vi "Reader kod10.vi"() -> ()   [LabVIEW 2021]
uses:
  <vilib>/Utility/file.llb/Write Delimited Spreadsheet (string).vi
  <vilib>/Utility/file.llb/Write Delimited Spreadsheet (DBL).vi
  <vilib>/FPGAPlugInAG/myRIO-1900/niLvFpga_Open_myRIO-1900.vi
  <vilib>/rvi/interface/common/dynamic/niFpgaDynamicAddResources.vi
  <vilib>/Utility/error.llb/Error Cluster From Error Code.vi
  <vilib>/rvi/errors/niLvFpgaAdjustHostInterfaceError.vi
  <vilib>/rvi/interface/nirviOpenFPGA/nirviOpenFPGA.xnode
  FPGA Bitfiles/projekt-bms10_FPGATarget_FPG10_wC+vpsaqoBo.lvbitx
  FPG10.vi
  <vilib>/rvi/interface/nirviReadWriteControl/nirviReadWriteControl.xnode
  <vilib>/rvi/interface/Simulation/niFpgaSimulationCallBeginRW.vi
  NiFpgaLv.dll
panel:
  out "Spänning 144 output 3":fxp<+/-,26,14>
  in  "stop 4":bool
  out "Loopar":fxp<+/-,64,32>
  out "SoC minus":fxp<+/-,32,16> format="%.21g"
  in  "stop 2":bool
  out "SoC":fxp<+/-,64,56>
  out "Batteri 2":fxp<+/-,64,54> format="%.21g"
  out "Ström 144 output":dbl format="%.2f"
  out "Spänning 144 output":fxp<+/-,64,50>
  out "x/y":fxp<+/-,49,33>
  out "PERIOD TIME [ms] 12":u32
  out "DUTY CYCLE [ticks] 12":u32
  out "duty cycle 12":dbl
  out "PERIOD TIME [ms] 11":u32
  out "DUTY CYCLE [ticks] 11":u32
  out "duty cycle 11":dbl
  out "PERIOD TIME [ms] 10":u32
  out "DUTY CYCLE [ticks] 10":u32
  out "duty cycle 6":dbl
  out "PERIOD TIME [ms] 9":u32
  out "DUTY CYCLE [ticks] 9":u32
  out "duty cycle 5":dbl
  out "PERIOD TIME [ms] 8":u32
  out "DUTY CYCLE [ticks] 8":u32
  out "duty cycle 10":dbl
  out "PERIOD TIME [ms] 7":u32
  out "DUTY CYCLE [ticks] 7":u32
  out "duty cycle 9":dbl
  out "PERIOD TIME [ms] 6":u32
  out "DUTY CYCLE [ticks] 6":u32
  out "duty cycle 4":dbl
  out "PERIOD TIME [ms] 5":u32
  out "DUTY CYCLE [ticks] 5":u32
  out "duty cycle 3":dbl
  out "PERIOD TIME [ms] 4":u32
  out "DUTY CYCLE [ticks] 4":u32
  out "duty cycle 8":dbl
  out "PERIOD TIME [ms] 3":u32
  out "DUTY CYCLE [ticks] 3":u32
  out "duty cycle 7":dbl
  out "PERIOD TIME [ms] 2":u32
  out "DUTY CYCLE [ticks] 2":u32
  out "duty cycle 2":dbl
  out "PERIOD TIME [ms]":u32
  out "DUTY CYCLE [ticks]":u32
  out "duty cycle":dbl format="%#.4f"
  in  "stop":bool
  out "appended array":dbl[][](array[numeric])
  in  "file path (dialog if empty)":path
  out "Array":string[](array[string])
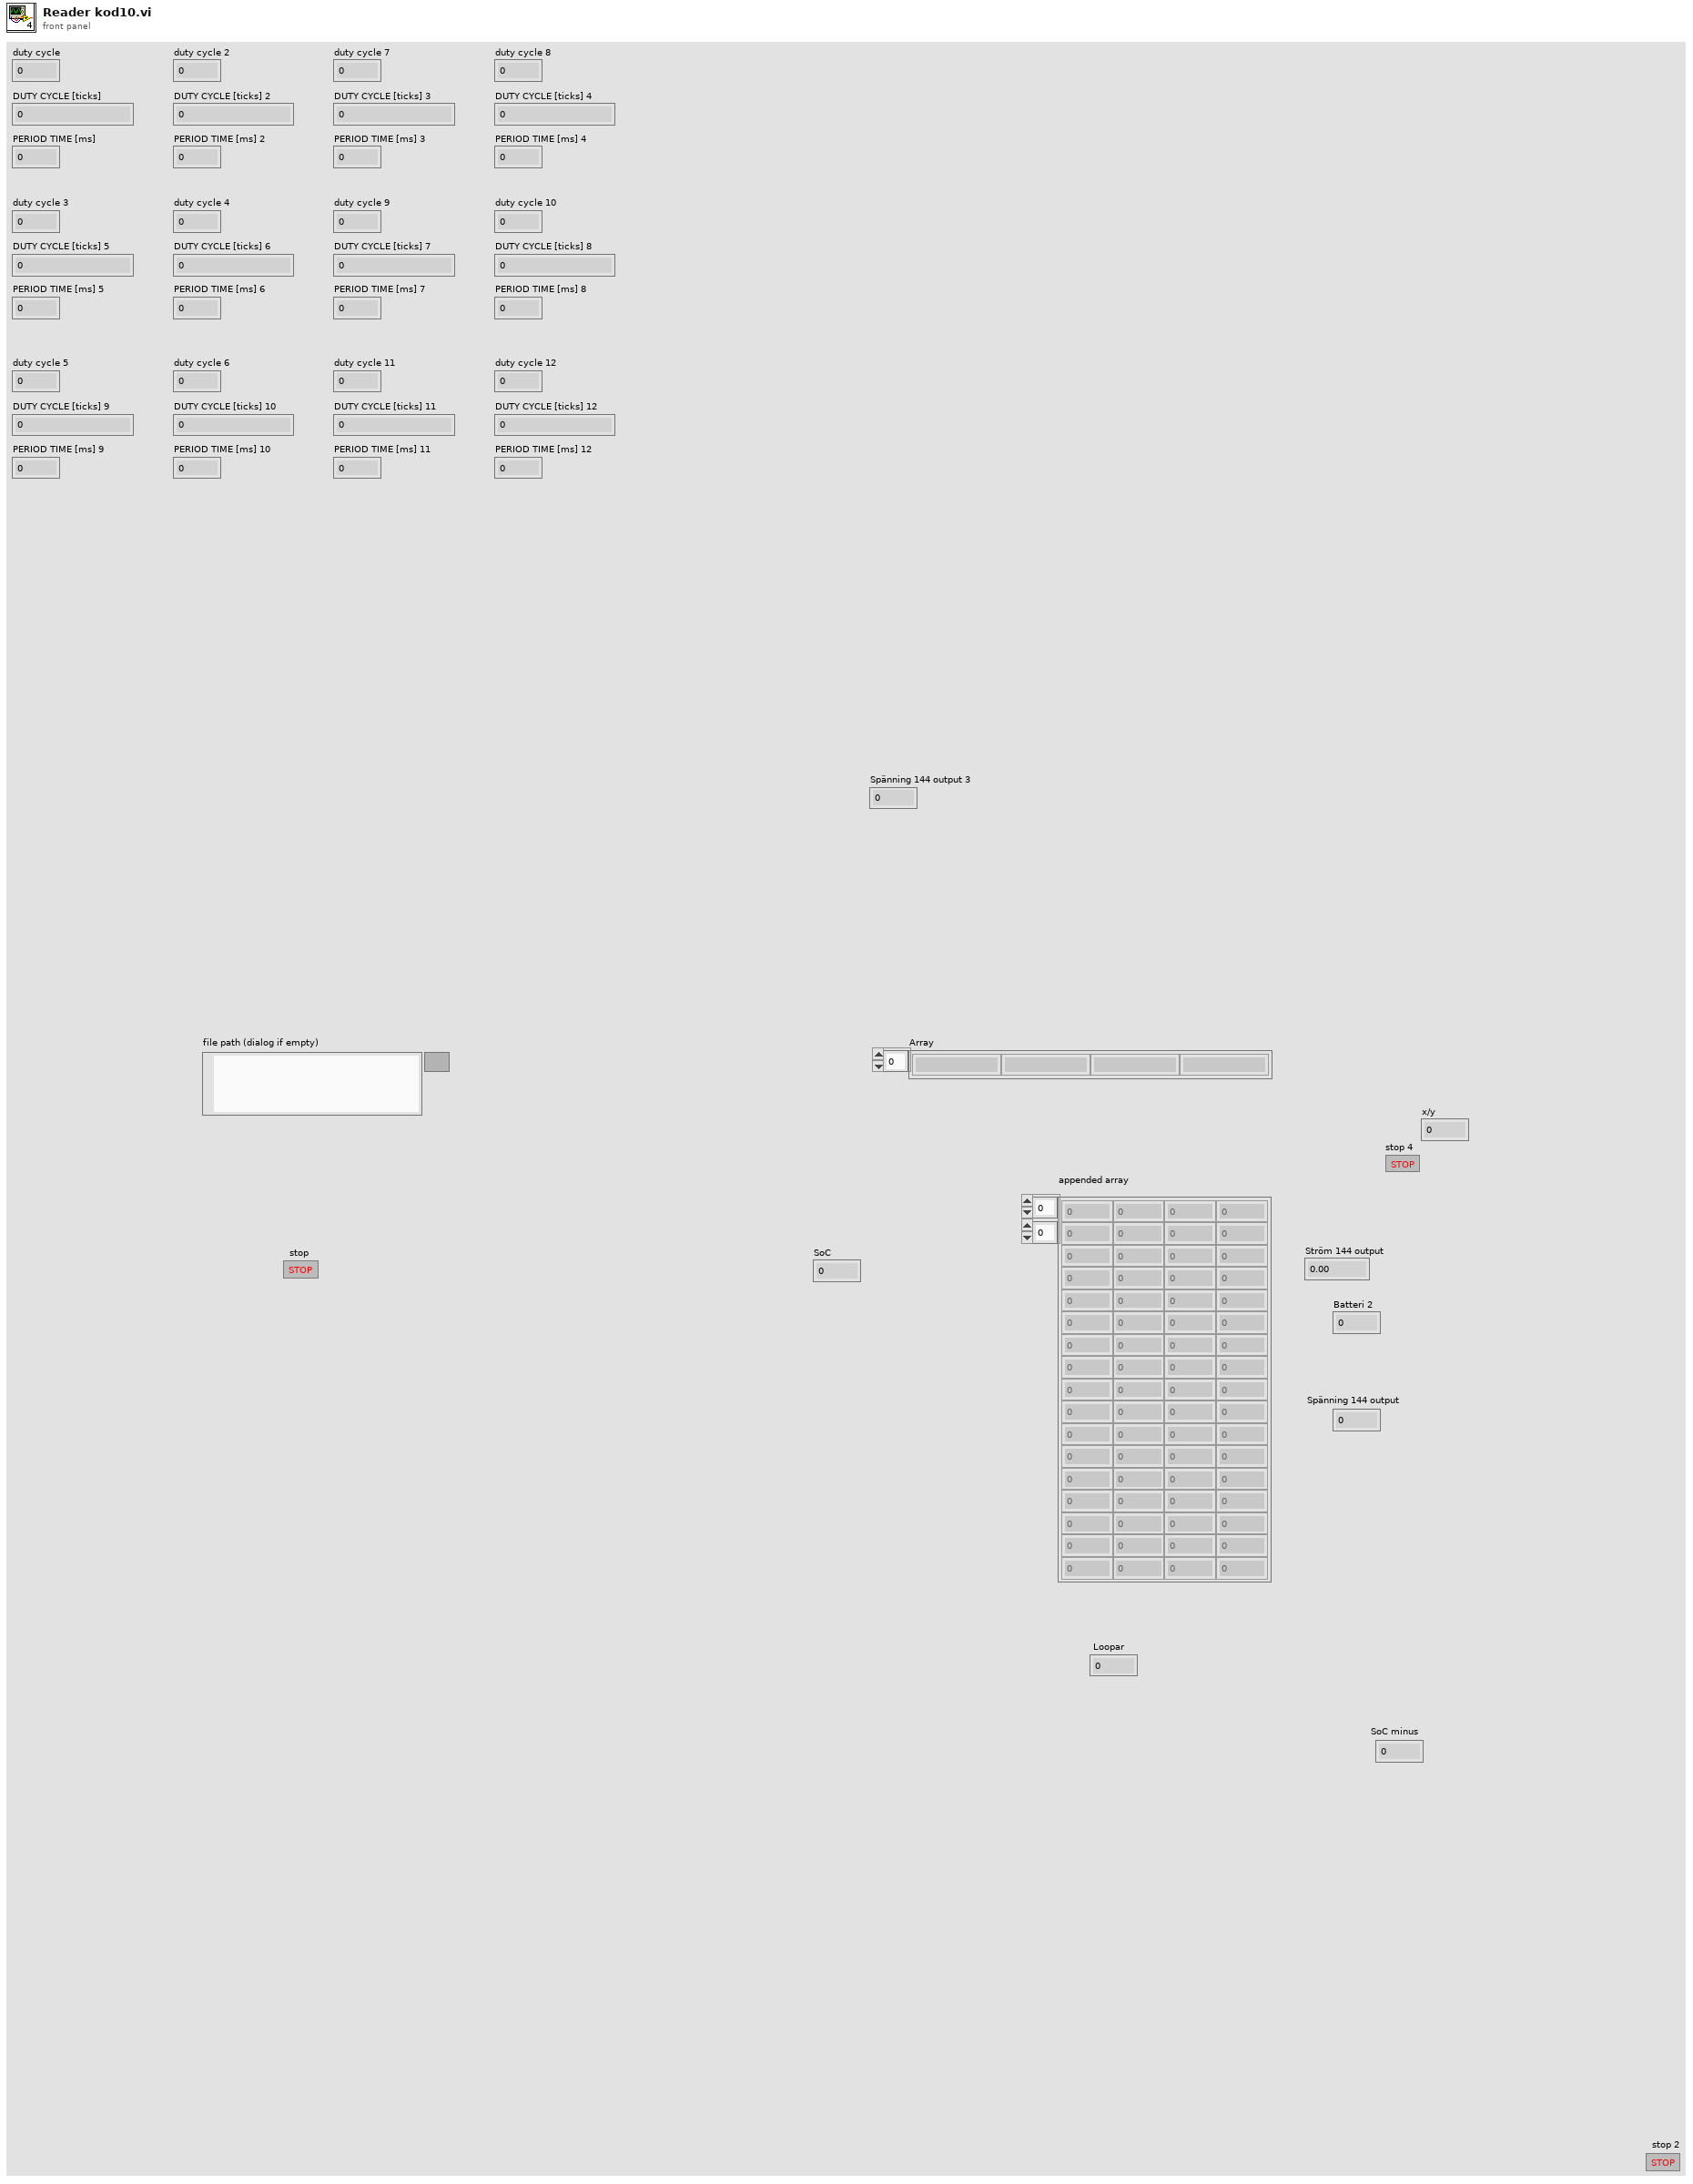
[diagram p1: front panel]
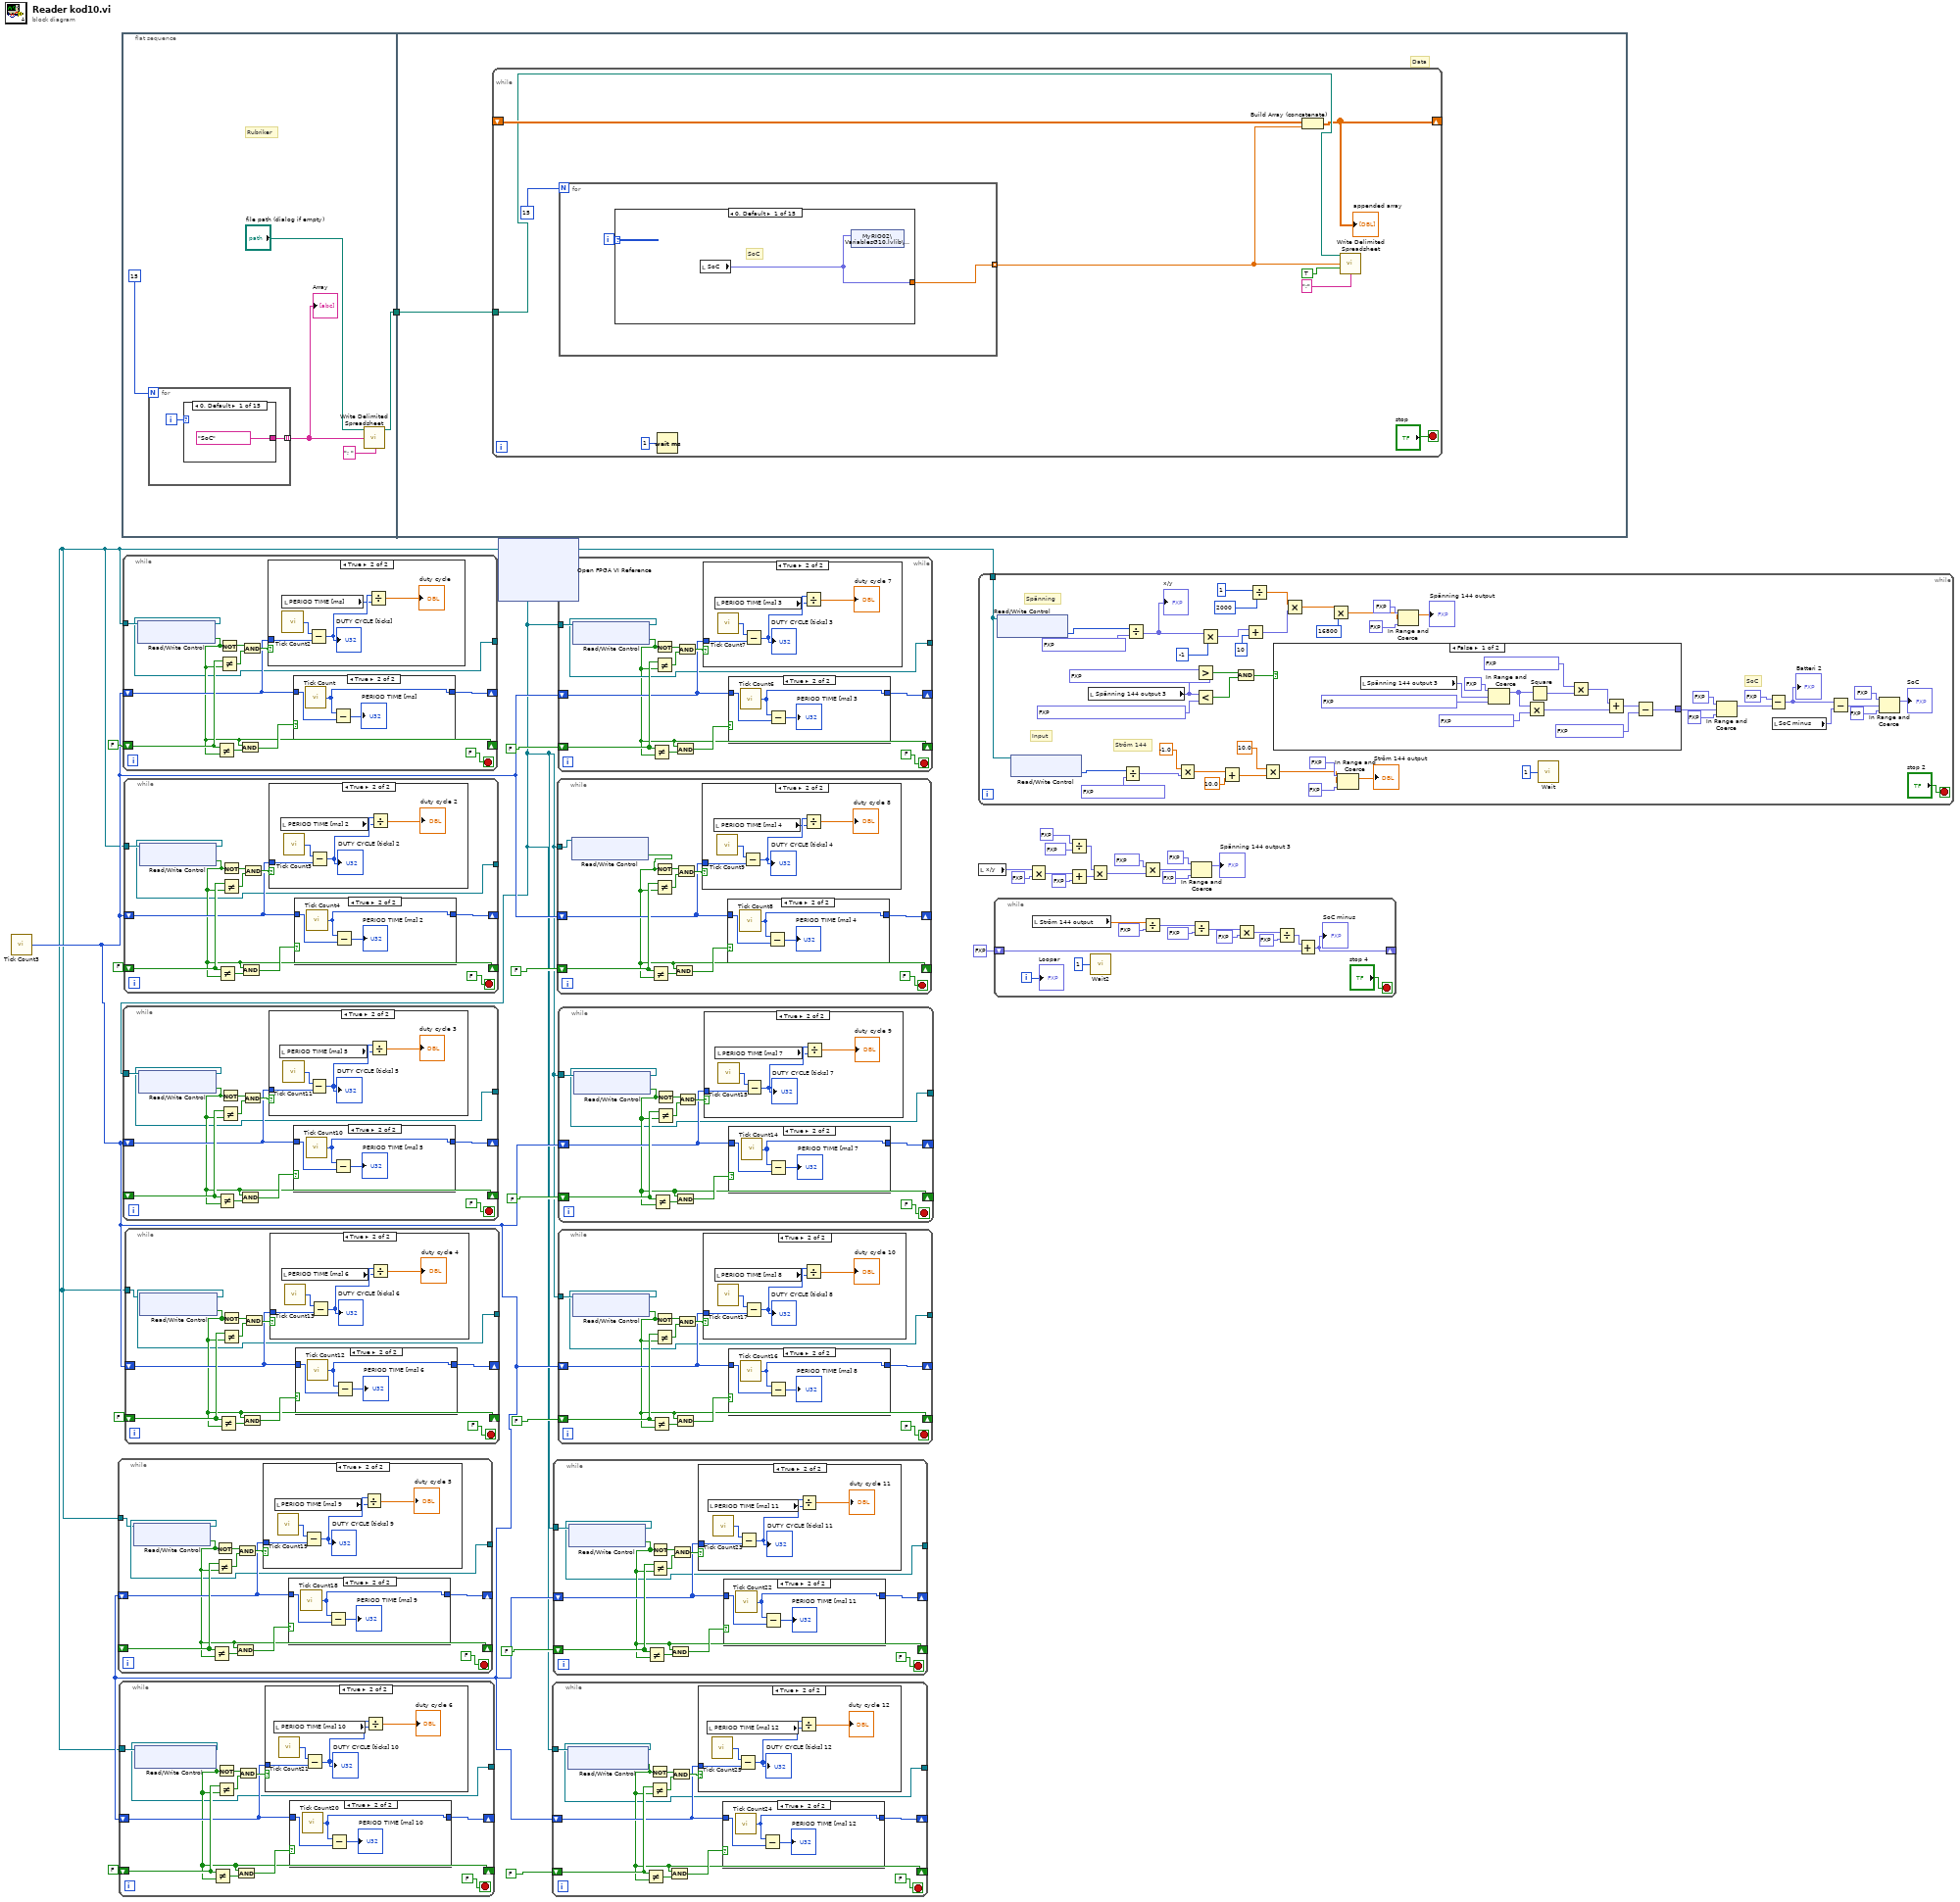
[diagram p0: block diagram]
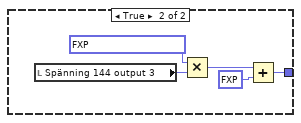
[diagram p2: hidden frame]
diagram:
  n1 = call "Tick Count3"() -> ("Tick Count(Ticks)"=w17:u32)
  n2 = flat-sequence {
    tunnel: [w29] -> w28
    tunnel: w28 -> [w51]
    frame #0 {
      # "Rubriker"
      n3 = for {
        N: 15 -> [_]
        tunnel: [w34] -> w33 mode=indexing
        i -> [w35]
        n4 = case shown="0, Default" w35 {
          tunnel: ["SoC" "Ström Högspänning" "Spänning 144" "Duty cycle" "Duty cycle 2" "Duty cycle 3" "Duty cycle 4" "Duty cycle 5" "Duty cycle 6" "Duty cycle 7" "Duty cycle 8" "Duty cycle 9" "Duty cycle 10" "Duty cycle 11" "Duty cycle 12"] -> w34
          frame 0, Default {
          }
          frame 1 {
          }
          frame 2 {
          }
          frame 3 {
          }
          frame 4 {
          }
          frame 5 {
          }
          frame 6 {
          }
          frame 7 {
          }
          frame 8 {
          }
          frame 9 {
          }
          frame 10 {
          }
          frame 11 {
          }
          frame 12 {
          }
          frame 13 {
          }
          frame 14 {
          }
        }
      }
      "Array" <- w33
      n5 = call-poly <vilib>:"Write Delimited Spreadsheet.vi"("file path (dialog if empty)"="file path (dialog if empty)", "1D data"=w33, "delimiter (\\t)"="; " ("delimiter (\\t)")) -> ("new file path (Not A Path if cancelled)"=w29:path)  [unwired: 11 in, 1 out]
    }
    frame #1 {
      # "Data"
      n6 = while {
        tunnel: w51 -> [w54]
        shift-right: [w52] -> _
        shift-left: _ -> [w56]
        stop <- "stop" stop-if-true
        n7 = for {
          N: 15 -> [_]
          tunnel: [w61] -> w53 mode=indexing
          i -> [w62]
          n8 = case shown="0, Default" w62 {
            tunnel: [w63 w64 w65 w66 w67 w68 w69 w70 w71 w72 w73 w74 w75 w76 w77] -> w61
            frame 0, Default {
              # "SoC"
              n9 = local read "SoC"() -> (w63:fxp<+/-,64,56>)
              n10 = shared-variable "MyRIO02\\VariablesG10.lvlib\\SoC10"(w63) -> ()  [unwired: 1 in, 1 out]
            }
            frame 1 {
              # "Ström 200 A"
              n11 = local read "Ström 144 output"() -> (w64:dbl)
            }
            frame 2 {
              # "Spänning 144"
              n12 = local read "Spänning 144 output"() -> (w65:fxp<+/-,64,50>)
            }
            frame 3 {
              n13 = local read "duty cycle"() -> (w66:dbl)
            }
            frame 4 {
              n14 = local read "duty cycle 2"() -> (w67:dbl)
            }
            frame 5 {
              n15 = local read "duty cycle 3"() -> (w68:dbl)
            }
            frame 6 {
              n16 = local read "duty cycle 4"() -> (w69:dbl)
            }
            frame 7 {
              n17 = local read "duty cycle 5"() -> (w70:dbl)
            }
            frame 8 {
              n18 = local read "duty cycle 6"() -> (w71:dbl)
            }
            frame 9 {
              n19 = local read "duty cycle 7"() -> (w72:dbl)
            }
            frame 10 {
              n20 = local read "duty cycle 8"() -> (w73:dbl)
            }
            frame 11 {
              n21 = local read "duty cycle 9"() -> (w74:dbl)
            }
            frame 12 {
              n22 = local read "duty cycle 10"() -> (w75:dbl)
            }
            frame 13 {
              n23 = local read "duty cycle 11"() -> (w76:dbl)
            }
            frame 14 {
              n24 = local read "duty cycle 12"() -> (w77:dbl)
            }
          }
        }
        n25 = Wait (ms)(milliseconds to wait=u32 1) -> ()  [unwired: 1 out]
        n26 = Build Array (concatenate)(w56, w53) -> (w52:dbl[][])
        "appended array" <- w52
        n27 = call-poly <vilib>:"Write Delimited Spreadsheet.vi"("file path (dialog if empty)"=w54, "1D data"=w53, "append to file? (new file:F)"=TRUE, "delimiter (\\t)"=";" ("delimiter (\\t)")) -> ()  [unwired: 10 in, 2 out]
      }
    }
  }
  n28 = xnode "Open FPGA VI Reference"() -> ("FPGA VI Reference Out"=w1:refnum<k20>)  [unwired: 2 in, 1 out]
  n29 = while {
    shift-right: [w80] -> _
    shift-left: _ -> [w83]
    shift-right: [w88] -> _
    shift-left: w17 -> [w81]
    tunnel: [w79] -> _
    tunnel: w1 -> [w78]
    stop <- FALSE stop-if-true
    n30 = xnode "Read/Write Control"("FPGA VI Reference In"=w78) -> ("FPGA VI Reference Out"=w79:refnum<k20>, "ConnectorA/DIO4"=w80:bool)  [unwired: 1 in, 1 out]
    n31 = Not Equal?(x=w83, y=w80) -> (x != y?=w87:bool)
    n32 = Not(x=w80) -> (.not. x?=w84:bool)
    n33 = Not Equal?(x=w83, y=w80) -> (x != y?=w85:bool)
    n34 = And(x=w80, y=w87) -> (x .and. y?=w86:bool)
    n35 = And(x=w84, y=w85) -> (x .and. y?=w82:bool)
    n36 = case shown="True" w82 {
      tunnel: w81 -> [_ w94]
      frame False {
      }
      frame True {
        n37 = local read "PERIOD TIME [ms] 9"() -> (w92:u32)
        n38 = call "Tick Count19"() -> ("Tick Count(Ticks)"=w91:u32)
        n39 = Subtract(x=w91, y=w94) -> (x-y=w93:u32)
        "DUTY CYCLE [ticks] 9" <- w93
        n40 = Divide(x=w93, y=w92) -> (x/y=→"duty cycle 5":dbl)
      }
    }
    n41 = case shown="True" w86 {
      tunnel: w81 -> [w95 w98]
      tunnel: [w95 w96] -> w88
      frame False {
      }
      frame True {
        n42 = call "Tick Count18"() -> ("Tick Count(Ticks)"=w96:u32)
        n43 = Subtract(x=w96, y=w98) -> (x-y=→"PERIOD TIME [ms] 9":u32)
      }
    }
  }
  n44 = while {
    shift-right: [w100] -> _
    shift-left: FALSE -> [w104]
    shift-right: [w109] -> _
    shift-left: w17 -> [w102]
    tunnel: w1 -> [w101]
    tunnel: [w99] -> _
    stop <- FALSE stop-if-true
    n45 = xnode "Read/Write Control"("FPGA VI Reference In"=w101) -> ("FPGA VI Reference Out"=w99:refnum<k20>, "ConnectorA/DIO13"=w100:bool)  [unwired: 1 in, 1 out]
    n46 = Not Equal?(x=w104, y=w100) -> (x != y?=w108:bool)
    n47 = Not(x=w100) -> (.not. x?=w105:bool)
    n48 = Not Equal?(x=w104, y=w100) -> (x != y?=w106:bool)
    n49 = And(x=w100, y=w108) -> (x .and. y?=w107:bool)
    n50 = And(x=w105, y=w106) -> (x .and. y?=w103:bool)
    n51 = case shown="True" w103 {
      tunnel: w102 -> [_ w115]
      frame False {
      }
      frame True {
        n52 = local read "PERIOD TIME [ms] 10"() -> (w113:u32)
        n53 = call "Tick Count21"() -> ("Tick Count(Ticks)"=w112:u32)
        n54 = Subtract(x=w112, y=w115) -> (x-y=w114:u32)
        "DUTY CYCLE [ticks] 10" <- w114
        n55 = Divide(x=w114, y=w113) -> (x/y=→"duty cycle 6":dbl)
      }
    }
    n56 = case shown="True" w107 {
      tunnel: w102 -> [w116 w119]
      tunnel: [w116 w117] -> w109
      frame False {
      }
      frame True {
        n57 = call "Tick Count20"() -> ("Tick Count(Ticks)"=w117:u32)
        n58 = Subtract(x=w117, y=w119) -> (x-y=→"PERIOD TIME [ms] 10":u32)
      }
    }
  }
  n59 = while {
    shift-right: [w121] -> _
    shift-left: FALSE -> [w125]
    shift-right: [w130] -> _
    shift-left: w17 -> [w123]
    tunnel: w1 -> [w122]
    tunnel: [w120] -> _
    stop <- FALSE stop-if-true
    n60 = xnode "Read/Write Control"("FPGA VI Reference In"=w122) -> ("FPGA VI Reference Out"=w120:refnum<k20>, "ConnectorA/DIO0"=w121:bool)  [unwired: 1 in, 1 out]
    n61 = Not Equal?(x=w125, y=w121) -> (x != y?=w129:bool)
    n62 = Not(x=w121) -> (.not. x?=w126:bool)
    n63 = Not Equal?(x=w125, y=w121) -> (x != y?=w127:bool)
    n64 = And(x=w121, y=w129) -> (x .and. y?=w128:bool)
    n65 = And(x=w126, y=w127) -> (x .and. y?=w124:bool)
    n66 = case shown="True" w124 {
      tunnel: w123 -> [_ w136]
      frame False {
      }
      frame True {
        n67 = local read "PERIOD TIME [ms]"() -> (w134:u32)
        n68 = call "Tick Count2"() -> ("Tick Count(Ticks)"=w133:u32)
        n69 = Subtract(x=w133, y=w136) -> (x-y=w135:u32)
        "DUTY CYCLE [ticks]" <- w135
        n70 = Divide(x=w135, y=w134) -> (x/y=→"duty cycle":dbl)
      }
    }
    n71 = case shown="True" w128 {
      tunnel: w123 -> [w137 w140]
      tunnel: [w137 w138] -> w130
      frame False {
      }
      frame True {
        n72 = call "Tick Count"() -> ("Tick Count(Ticks)"=w138:u32)
        n73 = Subtract(x=w138, y=w140) -> (x-y=→"PERIOD TIME [ms]":u32)
      }
    }
  }
  n74 = while {
    shift-right: [w142] -> _
    shift-left: _ -> [w146]
    shift-right: [w151] -> _
    shift-left: w17 -> [w144]
    tunnel: w1 -> [w143]
    tunnel: [w141] -> _
    stop <- FALSE stop-if-true
    n75 = xnode "Read/Write Control"("FPGA VI Reference In"=w143) -> ("FPGA VI Reference Out"=w141:refnum<k20>, "ConnectorA/DIO2"=w142:bool)  [unwired: 1 in, 1 out]
    n76 = Not Equal?(x=w146, y=w142) -> (x != y?=w150:bool)
    n77 = Not(x=w142) -> (.not. x?=w147:bool)
    n78 = Not Equal?(x=w146, y=w142) -> (x != y?=w148:bool)
    n79 = And(x=w142, y=w150) -> (x .and. y?=w149:bool)
    n80 = And(x=w147, y=w148) -> (x .and. y?=w145:bool)
    n81 = case shown="True" w145 {
      tunnel: w144 -> [_ w157]
      frame False {
      }
      frame True {
        n82 = local read "PERIOD TIME [ms] 5"() -> (w155:u32)
        n83 = call "Tick Count11"() -> ("Tick Count(Ticks)"=w154:u32)
        n84 = Subtract(x=w154, y=w157) -> (x-y=w156:u32)
        "DUTY CYCLE [ticks] 5" <- w156
        n85 = Divide(x=w156, y=w155) -> (x/y=→"duty cycle 3":dbl)
      }
    }
    n86 = case shown="True" w149 {
      tunnel: w144 -> [w158 w161]
      tunnel: [w158 w159] -> w151
      frame False {
      }
      frame True {
        n87 = call "Tick Count10"() -> ("Tick Count(Ticks)"=w159:u32)
        n88 = Subtract(x=w159, y=w161) -> (x-y=→"PERIOD TIME [ms] 5":u32)
      }
    }
  }
  n89 = while {
    shift-right: [w163] -> _
    shift-left: FALSE -> [w167]
    shift-right: [w172] -> _
    shift-left: w17 -> [w165]
    tunnel: w1 -> [w164]
    tunnel: [w162] -> _
    stop <- FALSE stop-if-true
    n90 = xnode "Read/Write Control"("FPGA VI Reference In"=w164) -> ("FPGA VI Reference Out"=w162:refnum<k20>, "ConnectorA/DIO1"=w163:bool)  [unwired: 1 in, 1 out]
    n91 = Not Equal?(x=w167, y=w163) -> (x != y?=w171:bool)
    n92 = Not(x=w163) -> (.not. x?=w168:bool)
    n93 = Not Equal?(x=w167, y=w163) -> (x != y?=w169:bool)
    n94 = And(x=w163, y=w171) -> (x .and. y?=w170:bool)
    n95 = And(x=w168, y=w169) -> (x .and. y?=w166:bool)
    n96 = case shown="True" w166 {
      tunnel: w165 -> [_ w178]
      frame False {
      }
      frame True {
        n97 = local read "PERIOD TIME [ms] 2"() -> (w176:u32)
        n98 = call "Tick Count5"() -> ("Tick Count(Ticks)"=w175:u32)
        n99 = Subtract(x=w175, y=w178) -> (x-y=w177:u32)
        "DUTY CYCLE [ticks] 2" <- w177
        n100 = Divide(x=w177, y=w176) -> (x/y=→"duty cycle 2":dbl)
      }
    }
    n101 = case shown="True" w170 {
      tunnel: w165 -> [w179 w182]
      tunnel: [w179 w180] -> w172
      frame False {
      }
      frame True {
        n102 = call "Tick Count4"() -> ("Tick Count(Ticks)"=w180:u32)
        n103 = Subtract(x=w180, y=w182) -> (x-y=→"PERIOD TIME [ms] 2":u32)
      }
    }
  }
  n104 = while {
    shift-right: [w185] -> _
    shift-left: FALSE -> [w188]
    shift-right: [w193] -> _
    shift-left: w17 -> [w186]
    tunnel: [w184] -> _
    tunnel: w1 -> [w183]
    stop <- FALSE stop-if-true
    n105 = xnode "Read/Write Control"("FPGA VI Reference In"=w183) -> ("FPGA VI Reference Out"=w184:refnum<k20>, "ConnectorA/DIO3"=w185:bool)  [unwired: 1 in, 1 out]
    n106 = Not Equal?(x=w188, y=w185) -> (x != y?=w192:bool)
    n107 = Not(x=w185) -> (.not. x?=w189:bool)
    n108 = Not Equal?(x=w188, y=w185) -> (x != y?=w190:bool)
    n109 = And(x=w185, y=w192) -> (x .and. y?=w191:bool)
    n110 = And(x=w189, y=w190) -> (x .and. y?=w187:bool)
    n111 = case shown="True" w187 {
      tunnel: w186 -> [_ w199]
      frame False {
      }
      frame True {
        n112 = local read "PERIOD TIME [ms] 6"() -> (w197:u32)
        n113 = call "Tick Count13"() -> ("Tick Count(Ticks)"=w196:u32)
        n114 = Subtract(x=w196, y=w199) -> (x-y=w198:u32)
        "DUTY CYCLE [ticks] 6" <- w198
        n115 = Divide(x=w198, y=w197) -> (x/y=→"duty cycle 4":dbl)
      }
    }
    n116 = case shown="True" w191 {
      tunnel: w186 -> [w200 w203]
      tunnel: [w200 w201] -> w193
      frame False {
      }
      frame True {
        n117 = call "Tick Count12"() -> ("Tick Count(Ticks)"=w201:u32)
        n118 = Subtract(x=w201, y=w203) -> (x-y=→"PERIOD TIME [ms] 6":u32)
      }
    }
  }
  n119 = while {
    shift-right: [w205] -> _
    shift-left: FALSE -> [w209]
    shift-right: [w214] -> _
    shift-left: w17 -> [w207]
    tunnel: w1 -> [w206]
    tunnel: [w204] -> _
    stop <- FALSE stop-if-true
    n120 = xnode "Read/Write Control"("FPGA VI Reference In"=w206) -> ("FPGA VI Reference Out"=w204:refnum<k20>, "ConnectorB/DIO13"=w205:bool)  [unwired: 1 in, 1 out]
    n121 = Not Equal?(x=w209, y=w205) -> (x != y?=w213:bool)
    n122 = Not(x=w205) -> (.not. x?=w210:bool)
    n123 = Not Equal?(x=w209, y=w205) -> (x != y?=w211:bool)
    n124 = And(x=w205, y=w213) -> (x .and. y?=w212:bool)
    n125 = And(x=w210, y=w211) -> (x .and. y?=w208:bool)
    n126 = case shown="True" w208 {
      tunnel: w207 -> [_ w220]
      frame False {
      }
      frame True {
        n127 = local read "PERIOD TIME [ms] 12"() -> (w218:u32)
        n128 = call "Tick Count25"() -> ("Tick Count(Ticks)"=w217:u32)
        n129 = Subtract(x=w217, y=w220) -> (x-y=w219:u32)
        "DUTY CYCLE [ticks] 12" <- w219
        n130 = Divide(x=w219, y=w218) -> (x/y=→"duty cycle 12":dbl)
      }
    }
    n131 = case shown="True" w212 {
      tunnel: w207 -> [w221 w224]
      tunnel: [w221 w222] -> w214
      frame False {
      }
      frame True {
        n132 = call "Tick Count24"() -> ("Tick Count(Ticks)"=w222:u32)
        n133 = Subtract(x=w222, y=w224) -> (x-y=→"PERIOD TIME [ms] 12":u32)
      }
    }
  }
  n134 = while {
    shift-right: [w226] -> _
    shift-left: FALSE -> [w230]
    shift-right: [w235] -> _
    shift-left: w17 -> [w228]
    tunnel: w1 -> [w227]
    tunnel: [w225] -> _
    stop <- FALSE stop-if-true
    n135 = xnode "Read/Write Control"("FPGA VI Reference In"=w227) -> ("FPGA VI Reference Out"=w225:refnum<k20>, "ConnectorB/DIO4"=w226:bool)  [unwired: 1 in, 1 out]
    n136 = Not Equal?(x=w230, y=w226) -> (x != y?=w234:bool)
    n137 = Not(x=w226) -> (.not. x?=w231:bool)
    n138 = Not Equal?(x=w230, y=w226) -> (x != y?=w232:bool)
    n139 = And(x=w226, y=w234) -> (x .and. y?=w233:bool)
    n140 = And(x=w231, y=w232) -> (x .and. y?=w229:bool)
    n141 = case shown="True" w229 {
      tunnel: w228 -> [_ w241]
      frame False {
      }
      frame True {
        n142 = local read "PERIOD TIME [ms] 11"() -> (w239:u32)
        n143 = call "Tick Count23"() -> ("Tick Count(Ticks)"=w238:u32)
        n144 = Subtract(x=w238, y=w241) -> (x-y=w240:u32)
        "DUTY CYCLE [ticks] 11" <- w240
        n145 = Divide(x=w240, y=w239) -> (x/y=→"duty cycle 11":dbl)
      }
    }
    n146 = case shown="True" w233 {
      tunnel: w228 -> [w242 w245]
      tunnel: [w242 w243] -> w235
      frame False {
      }
      frame True {
        n147 = call "Tick Count22"() -> ("Tick Count(Ticks)"=w243:u32)
        n148 = Subtract(x=w243, y=w245) -> (x-y=→"PERIOD TIME [ms] 11":u32)
      }
    }
  }
  n149 = while {
    shift-right: [w246] -> _
    shift-left: FALSE -> [w250]
    shift-right: [w255] -> _
    shift-left: w17 -> [w248]
    tunnel: w1 -> [w247]
    stop <- FALSE stop-if-true
    n150 = xnode "Read/Write Control"("FPGA VI Reference In"=w247) -> ("ConnectorB/DIO1"=w246:bool)  [unwired: 1 in, 2 out]
    n151 = Not Equal?(x=w250, y=w246) -> (x != y?=w254:bool)
    n152 = Not(x=w246) -> (.not. x?=w251:bool)
    n153 = Not Equal?(x=w250, y=w246) -> (x != y?=w252:bool)
    n154 = And(x=w246, y=w254) -> (x .and. y?=w253:bool)
    n155 = And(x=w251, y=w252) -> (x .and. y?=w249:bool)
    n156 = case shown="True" w249 {
      tunnel: w248 -> [_ w261]
      frame False {
      }
      frame True {
        n157 = local read "PERIOD TIME [ms] 4"() -> (w259:u32)
        n158 = call "Tick Count9"() -> ("Tick Count(Ticks)"=w258:u32)
        n159 = Subtract(x=w258, y=w261) -> (x-y=w260:u32)
        "DUTY CYCLE [ticks] 4" <- w260
        n160 = Divide(x=w260, y=w259) -> (x/y=→"duty cycle 8":dbl)
      }
    }
    n161 = case shown="True" w253 {
      tunnel: w248 -> [w262 w265]
      tunnel: [w262 w263] -> w255
      frame False {
      }
      frame True {
        n162 = call "Tick Count8"() -> ("Tick Count(Ticks)"=w263:u32)
        n163 = Subtract(x=w263, y=w265) -> (x-y=→"PERIOD TIME [ms] 4":u32)
      }
    }
  }
  n164 = while {
    shift-right: [w266] -> _
    shift-left: FALSE -> [w271]
    shift-right: [w276] -> _
    shift-left: w17 -> [w269]
    tunnel: w1 -> [w268]
    tunnel: [w267] -> _
    stop <- FALSE stop-if-true
    n165 = xnode "Read/Write Control"("FPGA VI Reference In"=w268) -> ("FPGA VI Reference Out"=w267:refnum<k20>, "ConnectorB/DIO0"=w266:bool)  [unwired: 1 in, 1 out]
    n166 = Not Equal?(x=w271, y=w266) -> (x != y?=w275:bool)
    n167 = Not(x=w266) -> (.not. x?=w272:bool)
    n168 = Not Equal?(x=w271, y=w266) -> (x != y?=w273:bool)
    n169 = And(x=w266, y=w275) -> (x .and. y?=w274:bool)
    n170 = And(x=w272, y=w273) -> (x .and. y?=w270:bool)
    n171 = case shown="True" w270 {
      tunnel: w269 -> [_ w282]
      frame False {
      }
      frame True {
        n172 = local read "PERIOD TIME [ms] 3"() -> (w280:u32)
        n173 = call "Tick Count7"() -> ("Tick Count(Ticks)"=w279:u32)
        n174 = Subtract(x=w279, y=w282) -> (x-y=w281:u32)
        "DUTY CYCLE [ticks] 3" <- w281
        n175 = Divide(x=w281, y=w280) -> (x/y=→"duty cycle 7":dbl)
      }
    }
    n176 = case shown="True" w274 {
      tunnel: w269 -> [w283 w286]
      tunnel: [w283 w284] -> w276
      frame False {
      }
      frame True {
        n177 = call "Tick Count6"() -> ("Tick Count(Ticks)"=w284:u32)
        n178 = Subtract(x=w284, y=w286) -> (x-y=→"PERIOD TIME [ms] 3":u32)
      }
    }
  }
  n179 = while {
    shift-right: [w288] -> _
    shift-left: FALSE -> [w292]
    shift-right: [w297] -> _
    shift-left: w17 -> [w290]
    tunnel: w1 -> [w289]
    tunnel: [w287] -> _
    stop <- FALSE stop-if-true
    n180 = xnode "Read/Write Control"("FPGA VI Reference In"=w289) -> ("FPGA VI Reference Out"=w287:refnum<k20>, "ConnectorB/DIO3"=w288:bool)  [unwired: 1 in, 1 out]
    n181 = Not Equal?(x=w292, y=w288) -> (x != y?=w296:bool)
    n182 = Not(x=w288) -> (.not. x?=w293:bool)
    n183 = Not Equal?(x=w292, y=w288) -> (x != y?=w294:bool)
    n184 = And(x=w288, y=w296) -> (x .and. y?=w295:bool)
    n185 = And(x=w293, y=w294) -> (x .and. y?=w291:bool)
    n186 = case shown="True" w291 {
      tunnel: w290 -> [_ w303]
      frame False {
      }
      frame True {
        n187 = local read "PERIOD TIME [ms] 8"() -> (w301:u32)
        n188 = call "Tick Count17"() -> ("Tick Count(Ticks)"=w300:u32)
        n189 = Subtract(x=w300, y=w303) -> (x-y=w302:u32)
        "DUTY CYCLE [ticks] 8" <- w302
        n190 = Divide(x=w302, y=w301) -> (x/y=→"duty cycle 10":dbl)
      }
    }
    n191 = case shown="True" w295 {
      tunnel: w290 -> [w304 w307]
      tunnel: [w304 w305] -> w297
      frame False {
      }
      frame True {
        n192 = call "Tick Count16"() -> ("Tick Count(Ticks)"=w305:u32)
        n193 = Subtract(x=w305, y=w307) -> (x-y=→"PERIOD TIME [ms] 8":u32)
      }
    }
  }
  n194 = while {
    shift-right: [w309] -> _
    shift-left: FALSE -> [w313]
    shift-right: [w318] -> _
    shift-left: w17 -> [w311]
    tunnel: w1 -> [w310]
    tunnel: [w308] -> _
    stop <- FALSE stop-if-true
    n195 = xnode "Read/Write Control"("FPGA VI Reference In"=w310) -> ("FPGA VI Reference Out"=w308:refnum<k20>, "ConnectorB/DIO2"=w309:bool)  [unwired: 1 in, 1 out]
    n196 = Not Equal?(x=w313, y=w309) -> (x != y?=w317:bool)
    n197 = Not(x=w309) -> (.not. x?=w314:bool)
    n198 = Not Equal?(x=w313, y=w309) -> (x != y?=w315:bool)
    n199 = And(x=w309, y=w317) -> (x .and. y?=w316:bool)
    n200 = And(x=w314, y=w315) -> (x .and. y?=w312:bool)
    n201 = case shown="True" w312 {
      tunnel: w311 -> [_ w324]
      frame False {
      }
      frame True {
        n202 = local read "PERIOD TIME [ms] 7"() -> (w322:u32)
        n203 = call "Tick Count15"() -> ("Tick Count(Ticks)"=w321:u32)
        n204 = Subtract(x=w321, y=w324) -> (x-y=w323:u32)
        "DUTY CYCLE [ticks] 7" <- w323
        n205 = Divide(x=w323, y=w322) -> (x/y=→"duty cycle 9":dbl)
      }
    }
    n206 = case shown="True" w316 {
      tunnel: w311 -> [w325 w328]
      tunnel: [w325 w326] -> w318
      frame False {
      }
      frame True {
        n207 = call "Tick Count14"() -> ("Tick Count(Ticks)"=w326:u32)
        n208 = Subtract(x=w326, y=w328) -> (x-y=→"PERIOD TIME [ms] 7":u32)
      }
    }
  }
  n209 = while {
    tunnel: w1 -> [w348]
    stop <- "stop 2" stop-if-true
    # "Input"
    # "Ström 144"
    # "SoC"
    # "Spänning"
    n210 = xnode "Read/Write Control"("FPGA VI Reference In"=w348) -> ("ConnectorC/AI1"=w349:i16)  [unwired: 1 in, 2 out]
    n211 = xnode "Read/Write Control"("FPGA VI Reference In"=w348) -> ("ConnectorC/AI0"=w347:i16)  [unwired: 1 in, 2 out]
    n212 = local read "Spänning 144 output 3"() -> (w358:fxp<+/-,26,14>)
    n213 = Divide(x=w347, y=fxp<+/-,32,16> 204.6999969482422) -> (x/y=w337:fxp<+/-,49,33>)
    n214 = Divide(x=w349, y=fxp<+/-,32,16> 204.6999969482422) -> (x/y=w344:fxp<+/-,49,33>)
    "x/y" <- w344
    n215 = Multiply(x=-1.0, y=w337) -> (x*y=w330:dbl)
    n216 = Greater?(x=w358, y=fxp<+/-,64,32> 109.33499999996275) -> (0:w356:bool)
    n217 = Less?(x=w358, y=fxp<+/-,64,32> 131.67700256337412) -> (x < y?=w357:bool)
    n218 = Multiply(x=w344, y=-1) -> (x*y=w333:fxp<+/-,64,64>)
    n219 = Add(x=w330, y=10.0) -> (x+y=w329:dbl)
    n220 = And(x=w356, y=w357) -> (x .and. y?=w362:bool)
    n221 = Add(x=w333, y=10) -> (x+y=w332:fxp<+/-,64,65>)
    n222 = Divide(x=1, y=2000) -> (x/y=w341:dbl)
    n223 = Multiply(x=10.0, y=w329) -> (x*y=w335:dbl)
    n224 = case shown="False" w362 {
      tunnel: [w381 w389] -> w361
      frame False {
        n225 = local read "Spänning 144 output 3"() -> (w378:fxp<+/-,26,14>)
        n226 = In Range and Coerce(upper limit=fxp<+,5,8> 168.0, x=w378, lower limit=fxp<+/-,64,32> 130.2269999999553) -> (coerced(x)=w377:fxp<+/-,64,32>)  [unwired: 1 out]
        n227 = Multiply(x=w377, y=fxp<+/-,32,16> 33.390350341796875) -> (x*y=w385:fxp<+/-,57,29>)
        n228 = Square(x=w377) -> (x^2=w388:fxp<+,49,25>)
        n229 = Multiply(x=fxp<+/-,32,16> -0.139373779296875, y=w388) -> (x*y=w386:fxp<+/-,64,42>)
        n230 = Add(x=w386, y=w385) -> (x+y=w383:fxp<+/-,64,44>)
        n231 = Subtract(x=w383, y=fxp<+/-,32,16> 1884.52197265625) -> (x-y=w381:fxp<+/-,64,46>)
      }
      frame True {
        n232 = local read "Spänning 144 output 3"() -> (w393:fxp<+/-,26,14>)
        n233 = Multiply(x=fxp<+/-,32,16> -0.1999969482421875, y=w393) -> (x*y=w391:fxp<+/-,57,29>)
        n234 = Add(x=w391, y=fxp<+,6,7> 122.0) -> (x+y=w389:fxp<+/-,57,29>)
      }
    }
    n235 = Multiply(x=w341, y=w332) -> (x*y=w340:dbl)
    n236 = Multiply(x=w340, y=16800) -> (x*y=w339:dbl)
    n237 = In Range and Coerce(upper limit=fxp<+,7,8> 250.0, x=w335, lower limit=fxp<+,1,1> 0.0) -> (coerced(x)=→"Ström 144 output":dbl)  [unwired: 1 out]
    n238 = In Range and Coerce(upper limit=fxp<+,5,8> 168.0, x=w339, lower limit=fxp<+,1,1> 0.0) -> (coerced(x)=→"Spänning 144 output":dbl)  [unwired: 1 out]
    n239 = call "Wait"("Count(mSec)"=u32 1) -> ()  [unwired: 1 out]
    n240 = In Range and Coerce(upper limit=fxp<+,5,7> 100.0, x=w361, lower limit=fxp<+,1,1> 0.0) -> (coerced(x)=w371:fxp<+/-,64,46>)  [unwired: 1 out]
    n241 = Subtract(x=fxp<+,5,7> 100.0, y=w371) -> (x-y=w369:fxp<+/-,64,54>)
    "Batteri 2" <- w369
    n242 = local read "SoC minus"() -> (w365:fxp<+/-,32,16>)
    n243 = Subtract(x=w369, y=w365) -> (x-y=w353:fxp<+/-,64,56>)
    n244 = In Range and Coerce(upper limit=fxp<+,5,7> 100.0, x=w353, lower limit=fxp<+,1,1> 0.0) -> (coerced(x)=→"SoC":fxp<+/-,64,56>)  [unwired: 1 out]
  }
  n245 = local read "x/y"() -> (w2:fxp<+/-,49,33>)
  n246 = while {
    shift-right: [w394] -> _
    shift-left: fxp<+/-,32,16> 0.0 -> [w401]
    i -> [w406]
    stop <- "stop 4" stop-if-true
    n247 = local read "Ström 144 output"() -> (w402:dbl)
    n248 = call "Wait2"("Count(mSec)"=u32 1) -> ()  [unwired: 1 out]
    n249 = Divide(x=w402, y=fxp<+,7,10> 1000.0) -> (x/y=w404:fxp<+/-,64,32>)
    n250 = Divide(x=w404, y=fxp<+,8,12> 3600.0) -> (x/y=w397:fxp<+/-,64,22>)
    n251 = Multiply(x=w397, y=fxp<+/-,32,16> 100.0) -> (x*y=w396:fxp<+/-,64,39>)
    n252 = Divide(x=w396, y=fxp<+,4,6> 60.0) -> (x/y=w395:fxp<+/-,64,35>)
    n253 = Add(x=w395, y=w401) -> (x+y=w394:fxp<+/-,32,16>)
    "SoC minus" <- w394
    "Loopar" <- w406
  }
  n254 = Multiply(x=w2, y=fxp<+/-,1,1> -1.0) -> (x*y=w7:fxp<+/-,16,10>)
  n255 = Divide(x=fxp<+,1,1> 1.0, y=fxp<+,7,11> 2000.0) -> (x/y=w10:fxp<+,1,-10>)
  n256 = Add(x=w7, y=fxp<+,3,4> 10.0) -> (x+y=w5:fxp<+/-,17,11>)
  n257 = Multiply(x=w10, y=w5) -> (x*y=w9:fxp<+/-,17,0>)
  n258 = Multiply(x=fxp<+,10,15> 16800.0, y=w9) -> (x*y=w13:fxp<+/-,26,14>)
  n259 = In Range and Coerce(upper limit=fxp<+,5,8> 168.0, x=w13, lower limit=fxp<+,1,1> 0.0) -> (coerced(x)=→"Spänning 144 output 3":fxp<+/-,26,14>)  [unwired: 1 out]
